vi "FTW-SQLite-RandomBLOB.vi"(0 "Number of Bytes":i32=1024, 11 "error in":errorcluster) -> (4 "Random BLOB":string, 15 "error out":errorcluster)   [LabVIEW 2015]
panel:
  # "Inputs"
  # "Outputs"
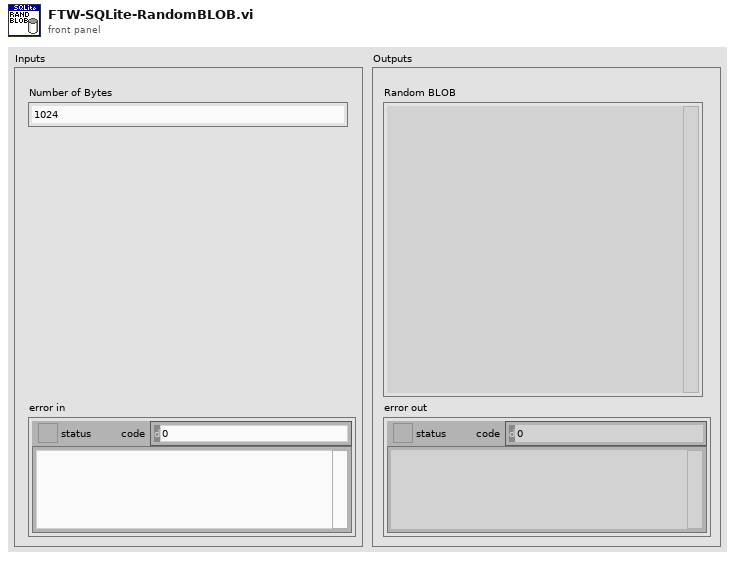
[diagram p1: front panel]
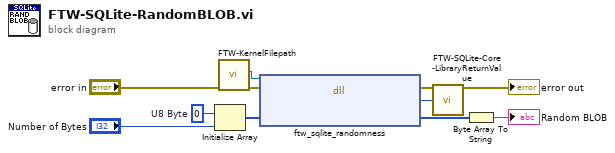
[diagram p0: block diagram]
diagram:
  w5 = u8 0  # U8 Byte
  n1 = Initialize Array(w5, "Number of Bytes") -> (w6:u8[])
  n2 = call "FTW-KernelFilepath.vi"("error in"="error in") -> ("error out"=w2:errorcluster, "Library Filepath"=w1:path)  [unwired: 8 in, 1 out]
  n3 = dll-call lib="?" fn="ftw_sqlite_randomness"(path in=w1, error in=w2, "Random Bytes Buffer"=w6) -> (error out=w11:errorcluster, "Return Value"=w10:i32, "Random Bytes Buffer"=w8:u8[])  [unwired: 1 in, 1 out]
  n4 = call "FTW-SQLite-Core-LibraryReturnValue.vi"("error in"=w11, "Return Value"=w10) -> ("error out"=→"error out":errorcluster)  [unwired: 13 in]
  n5 = Byte Array To String(unsigned byte array=w8) -> (string=→"Random BLOB":string)
